vi "Save Accel Data.vi"(0 "Accel Values":dbl[][](array[numeric])=[[1.0, 2.0, 3.0], [4.0, 5.0, 6.0], [7.0, 8.0, 9.0]], 11 "Error In":errorcluster) -> (4 "Pass?":bool, 6 "Pass/Fail #":i32)   [LabVIEW 2015]
uses:
  <vilib>/addons/_office/excel.llb/Excel Easy Table (num).vi
  <vilib>/Utility/NIReport.llb/NI_report.lvclass
  <vilib>/addons/_office/NI_ReportGenerationToolkit.lvlib
  <vilib>/Utility/NIReport.llb/Excel/NI_Excel.lvclass
panel:
  out "error out":errorcluster
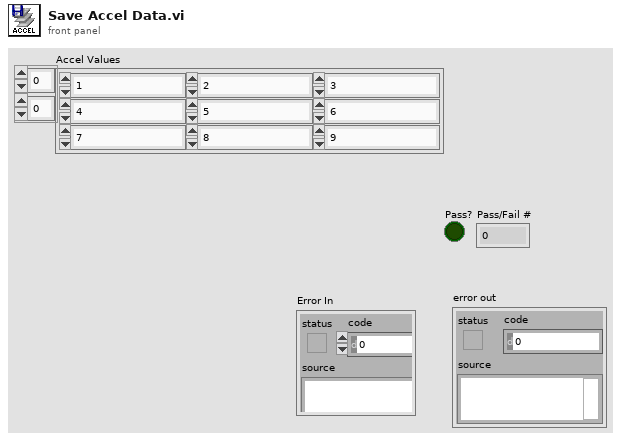
[diagram p1: front panel]
types:
  T1 = enum16{"maximized", "minimized", "normal", "no change"}
  T2 = enum16{"Standard Report", "HTML", "Word", "Excel"}
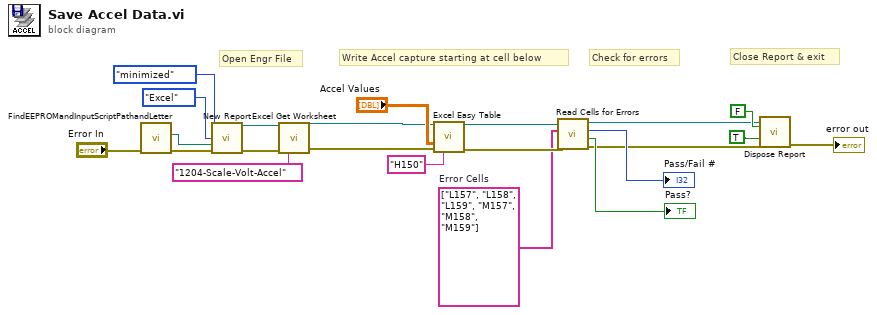
[diagram p0: block diagram]
diagram:
  w6 = string[] ["L157", "L158", "L159", "M157", "M158", "M159"]  # Error Cells
  # "Check for errors"
  # "Write Accel capture starting at cell below"
  # "Open Engr File"
  # "Close Report & exit"
  n1 = call "FindEEPROMandInputScriptPathandLetter.vi"("Error In"="Error In") -> ("Error Out"=w14:errorcluster, "Engr Result Path"=w22:path)  [unwired: 6 in, 1 out]
  n2 = call <vilib>:"New Report.vi"("window state (normal)"=T1."minimized", "report type"=T2."Excel", "template (empty)"=w22, "error in (no error)"=w14) -> ("report out"=w12:refnum<class "NI_report.lvclass">, "error out"=w13:errorcluster)  [unwired: 10 in]
  n3 = call <vilib>:"Excel Get Worksheet.vi"("report in"=w12, "error in (no error)"=w13, "name (\"\")"="1204-Scale-Volt-Accel" ("name (\"\")")) -> ("report out"=w11:refnum<class "NI_report.lvclass">, "error out"=w10:errorcluster)  [unwired: 11 in]
  n4 = call-poly <vilib>:"Excel Easy Table.vi"("report in"=w11, "text data"="Accel Values", "error in (no error)"=w10, "name (\"\")"="H150" ("name (\"\")")) -> ("report out"=w8:refnum<class "NI_report.lvclass">, "error out"=w7:errorcluster)  [unwired: 7 in, 3 out]
  n5 = call "Read Cells for Errors.vi"("error in (no error)"=w7, "Error Cells (ex:A12)"=w6, "NI_report in"=w8) -> ("error out"=w2:errorcluster, "Pass?"=→"Pass?":bool, "Error Code"=→"Pass/Fail #":i32, "NI_report out"=w3:refnum<class "NI_report.lvclass">)  [unwired: 5 in]
  n6 = call-dynamic "Dispose Report.vi"("report in"=w3, "wait until printing completed? (T)"=FALSE, "save changes? (F)"=TRUE, "error in (no error)"=w2) -> ("error out"=→"error out":errorcluster)  [unwired: 11 in]
